vi "ReadPatternFile.vi"(0 "PatternsXMLFileIn":path, 1 "PatternXMLFileContent":string, 5 "error in (no error)":errorcluster) -> (14 "Pattern":T3={"Version"="", "ID"="State", "Name"="State", "Category"="Behavioral", "Help"="State.htm", "Desc"="Allow an object to alter its behavior when its internal state changes. The object will appear to change its class."}, 15 "Nodes":T4[](array[typedef])=[{"ID"="Context", "Type"=enum."Class", "Name"="Context", "Stereotype"="", "X"=0, "Y"=0, "TypeSpecificData"=variant(cluster{"Attributes":cluster{"ID":string, "Name":string}[], "Methods":cluster{"ID":string, "Name":string}[]} {"Attributes"=[{"ID"="StateRef", "Name"="CurrentState : State"}], "Methods"=[{"ID"="Request", "Name"="Request()"}]})}, {"ID"="State", "Type"=enum."Class", "Name"="State", "Stereotype"="ABSTRACT", "X"=0, "Y"=0, "TypeSpecificData"=variant(cluster{"Attributes":cluster{"ID":string, "Name":string}[], "Methods":cluster{"ID":string, "Name":string}[]} {"Attributes"=[], "Methods"=[{"ID"="Handle", "Name"="Handle()"}]})}, {"ID"="ConcreteStateA", "Type"=enum."Class", "Name"="ConcreteStateA", "Stereotype"="", "X"=0, "Y"=0, "TypeSpecificData"=variant(cluster{"Attributes":cluster{"ID":string, "Name":string}[], "Methods":cluster{"ID":string, "Name":string}[]} {"Attributes"=[], "Methods"=[{"ID"="Handle", "Name"="Handle()"}]})}, {"ID"="ConcreteStateB", "Type"=enum."Class", "Name"="ConcreteStateB", "Stereotype"="", "X"=0, "Y"=0, "TypeSpecificData"=variant(cluster{"Attributes":cluster{"ID":string, "Name":string}[], "Methods":cluster{"ID":string, "Name":string}[]} {"Attributes"=[], "Methods"=[{"ID"="Handle", "Name"="Handle()"}]})}, {"ID"="RequestNote", "Type"=enum."Note", "Name"="", "Stereotype"="", "X"=0, "Y"=0, "TypeSpecificData"=variant(cluster{"Text":string, "Links":cluster{"ID":string, "source":string}[]} {"Text"="state->Handle()", "Links"=[{"ID"="ToRequest", "source"="Request"}]})}], 16 "Links":T1[](array[typedef])=[{"ID"="Aggregation", "Type"=enum."Aggregation", "Name"="", "StartText"="state", "EndText"="", "From"="Context", "To"="State"}], 17 "Valid":bool, 19 "error out":errorcluster)   [LabVIEW 2014]
uses:
  <resource>/Framework/Providers/Open_GDS/UML/DesignPattern/SubVIs/DesignPatterns_Node.ctl
  <resource>/Framework/Providers/Open_GDS/UML/DesignPattern/SubVIs/DesignPatterns_NodeType.ctl
  <resource>/Framework/Providers/Open_GDS/UML/DesignPattern/SubVIs/DesignPatterns_Pattern.ctl
  <resource>/Framework/Providers/Open_GDS/UML/DesignPattern/SubVIs/DesignPatterns_Link.ctl
  <resource>/Framework/Providers/Open_GDS/UML/DesignPattern/SubVIs/DesignPatterns_LinkType.ctl
  <resource>/Framework/Providers/Open_GDS/UML/DesignPattern/SubVIs/DesignPatterns_ClassNodeData.ctl
  <resource>/Framework/Providers/Open_GDS/UML/DesignPattern/SubVIs/DesignPatterns_Attribute.ctl
  <resource>/Framework/Providers/Open_GDS/UML/DesignPattern/SubVIs/DesignPatterns_Method.ctl
  <resource>/Framework/Providers/Open_GDS/UML/DesignPattern/SubVIs/DesignPatterns_InterfaceNodeData.ctl
  <resource>/Framework/Providers/Open_GDS/UML/DesignPattern/SubVIs/DesignPatterns_NoteNodeData.ctl
  <resource>/Framework/Providers/Open_GDS/UML/DesignPattern/SubVIs/DesignPatterns_NoteLink.ctl
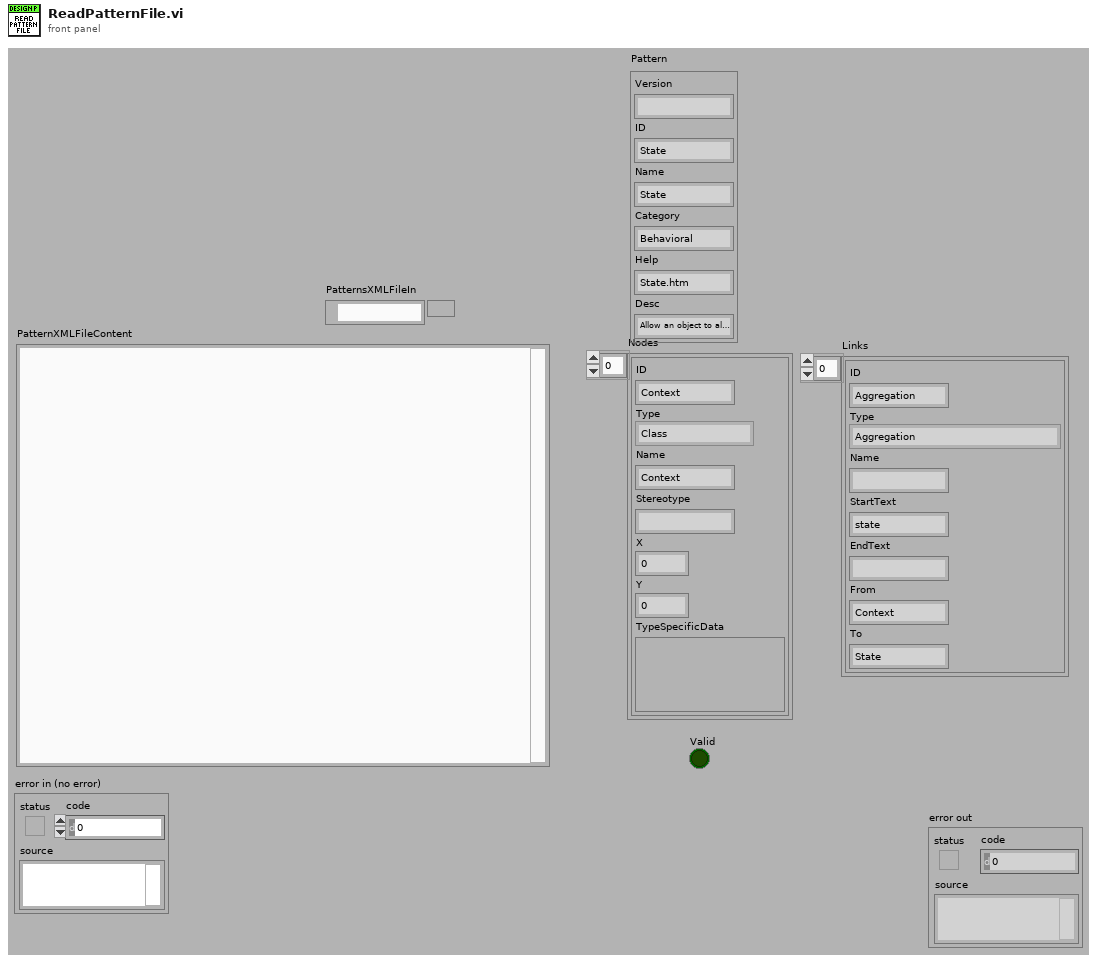
[diagram p1: front panel]
types:
  T1 = typedef "DesignPatterns_Link.ctl" = cluster{"ID":string, "Type":T2, "Name":string, "StartText":string, "EndText":string, "From":string, "To":string}
  T2 = typedef "DesignPatterns_LinkType.ctl" = enum16{"Dependency", "Inheritance", "Interface", "Association", "Aggregation", "CompositeAggregation"}
  T3 = typedef "DesignPatterns_Pattern.ctl" = cluster{"Version":string, "ID":string, "Name":string, "Category":string, "Help":string, "Desc":string}
  T4 = typedef "DesignPatterns_Node.ctl" = cluster{"ID":string, "Type":T5, "Name":string, "Stereotype":string, "X":i32, "Y":i32, "TypeSpecificData":variant}
  T5 = typedef "DesignPatterns_NodeType.ctl" = enum16{"Class", "Interface", "Note", "Package"}
  T6 = cluster{"Text":string, "Valid":bool, "Pattern":T3, "Nodes":T4[], "Links":T1[]}
  T7 = typedef "DesignPatterns_ClassNodeData.ctl" = cluster{"Description":string, "Attributes":T8[], "Methods":T9[]}
  T8 = typedef "DesignPatterns_Attribute.ctl" = cluster{"ID":string, "Name":string}
  T9 = typedef "DesignPatterns_Method.ctl" = cluster{"ID":string, "Name":string}
  T10 = typedef "DesignPatterns_InterfaceNodeData.ctl" = cluster{"Methods":T9[]}
  T11 = typedef "DesignPatterns_NoteNodeData.ctl" = cluster{"Text":string, "Links":T12[]}
  T12 = typedef "DesignPatterns_NoteLink.ctl" = cluster{"ID":string, "source":string}
  T13 = cluster{"id":string, "node.type":T5, "link.type":T2, "name":string, "stereotype":string, "X":i32, "Y":i32, "starttext":string, "endtext":string, "from":string, "to":string, "version":string, "category":string, "help":string}
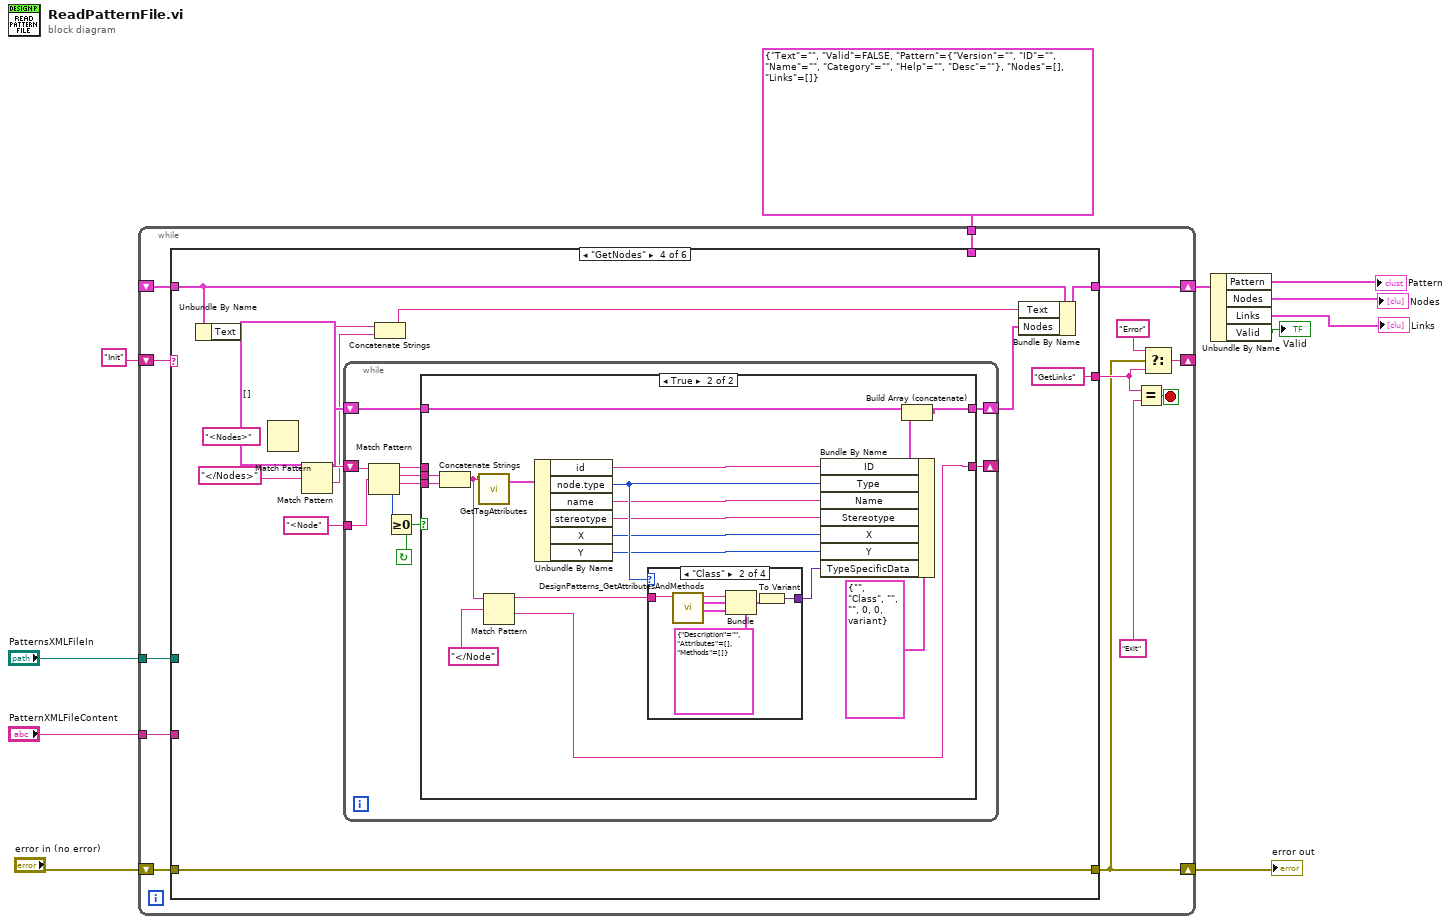
[diagram p0: block diagram]
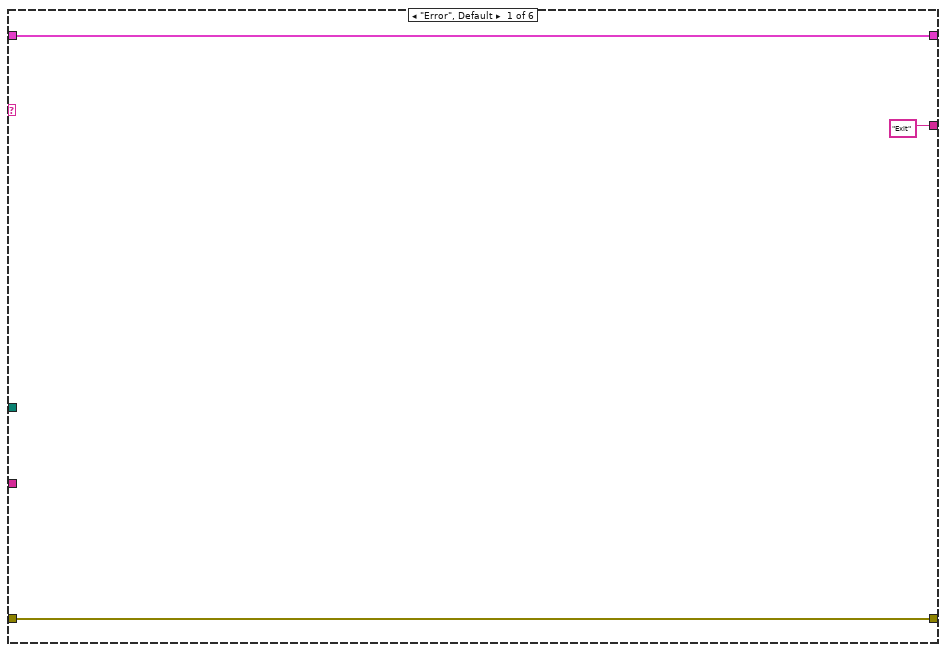
[diagram p2: hidden frame]
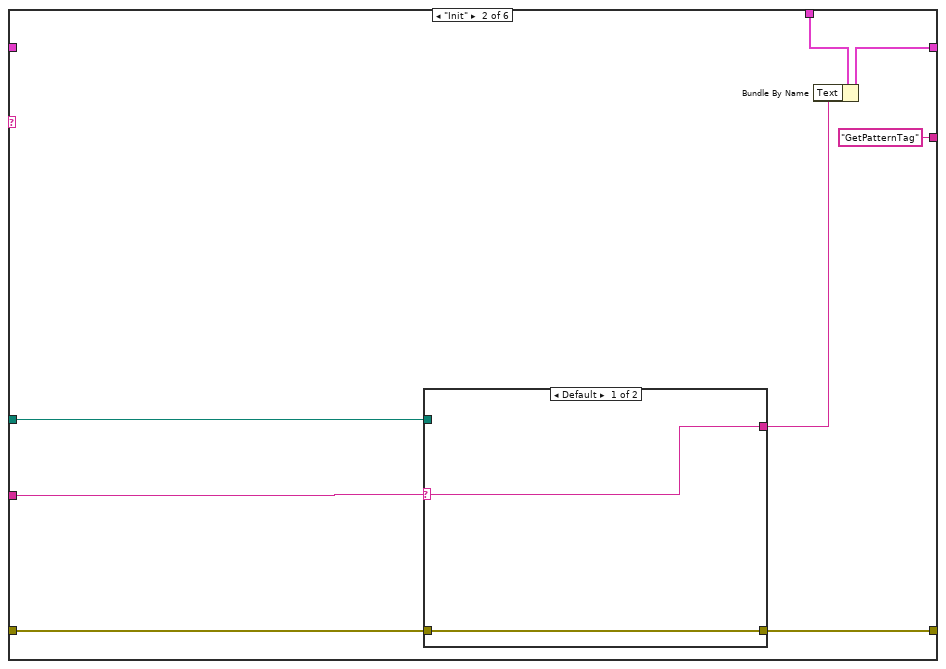
[diagram p3: hidden frame]
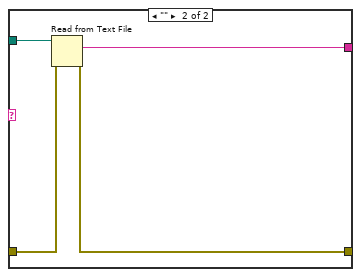
[diagram p4: hidden frame]
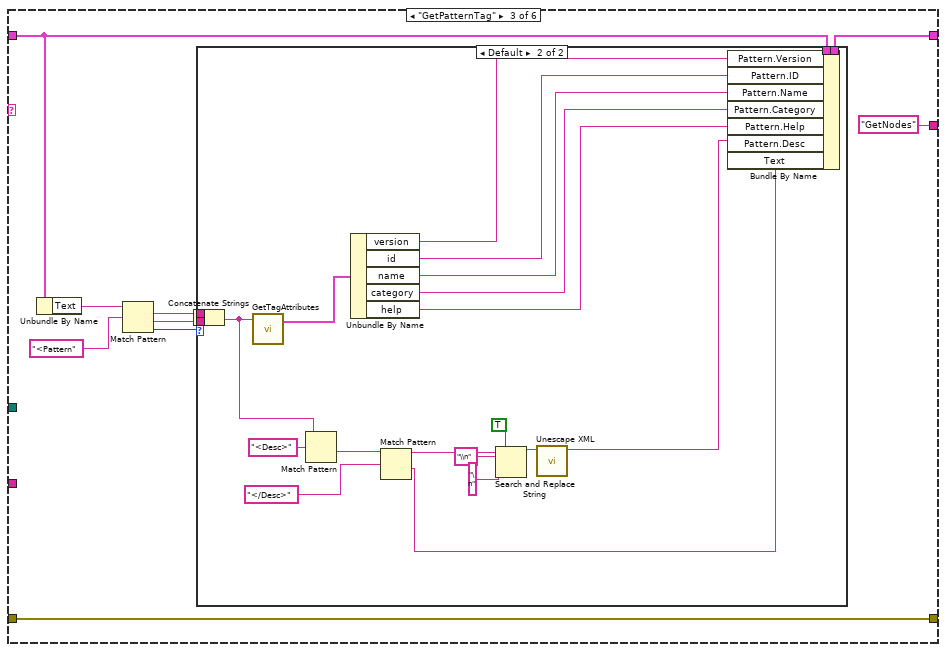
[diagram p5: hidden frame]
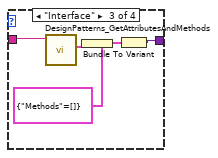
[diagram p9: hidden frame]
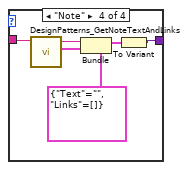
[diagram p10: hidden frame]
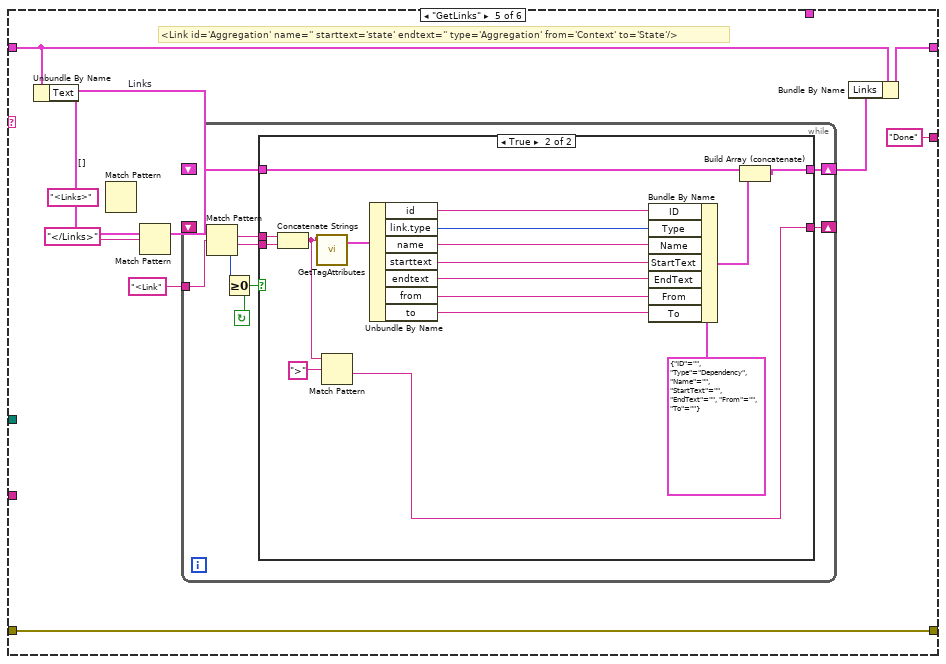
[diagram p11: hidden frame]
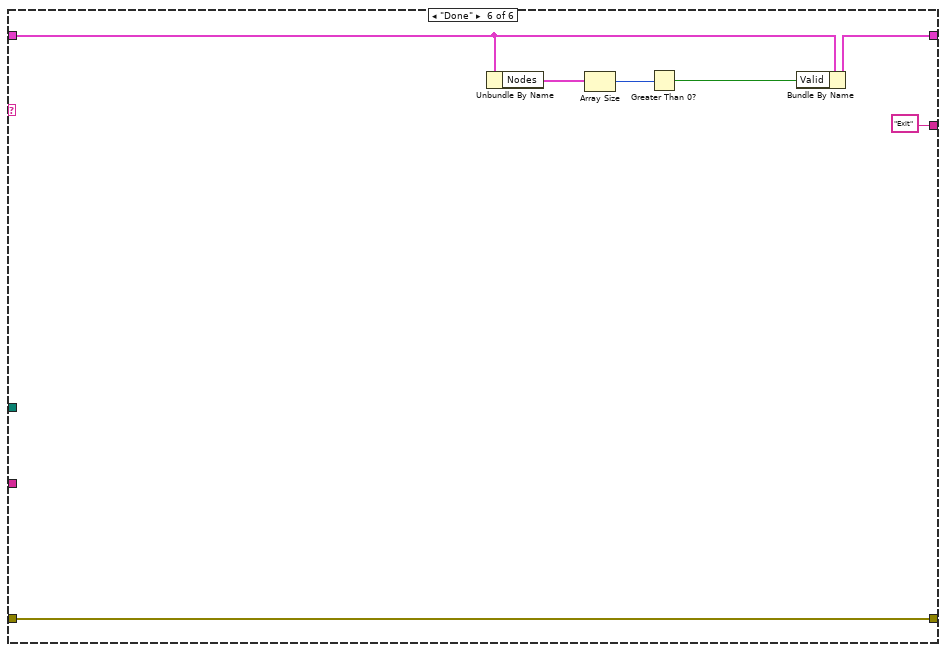
[diagram p13: hidden frame]
diagram:
  n1 = while {
    shift-right: [w17] -> w8
    shift-left: "error in (no error)" -> [w24]
    shift-right: [w22] -> _
    shift-left: "Init" -> [w23]
    shift-right: [w16] -> w11
    shift-left: _ -> [w15]
    tunnel: "PatternsXMLFileIn" -> [w14]
    tunnel: "PatternXMLFileContent" -> [w13]
    tunnel: T6 {"Text"="", "Valid"=FALSE, "Pattern"={"Version"="", "ID"="", "Name"="", "Category"="", "Help"="", "Desc"=""}, "Nodes"=[], "Links"=[]} -> [w12]
    stop <- w21 stop-if-true
    n2 = case shown="\"GetNodes\"" w23 {
      tunnel: w24 -> [w27 w32 w49 w87 w146 w174]
      tunnel: [w27 w31 w49 w87 w146 w174] -> w17
      tunnel: ["Exit" "GetPatternTag" "GetNodes" "GetLinks" "Done" "Exit"] -> w18
      tunnel: [w25 w29 w48 w79 w138 w180] -> w16
      tunnel: w15 -> [w25 _ w47 w80 w139 w179]
      tunnel: w14 -> [_ w33 _ _ _ _]
      tunnel: w13 -> [_ w34 _ _ _ _]
      tunnel: w12 -> [_ w30 _ _ _ _]
      frame "Error", Default {
      }
      frame "Init" {
        n3 = case shown="Default" w34 {
          selector: w34 -> [w36 _]
          tunnel: w33 -> [_ w41]
          tunnel: w32 -> [w37 w40]
          tunnel: [w37 w39] -> w31
          tunnel: [w36 w38] -> w28
          frame Default {
          }
          frame "" {
            n4 = Read from Text File(file (use dialog)=w41, error in=w40) -> (text=w38:string, error out=w39:errorcluster)  [unwired: 4 out]
          }
        }
        n5 = Bundle By Name(cluster=w30, "Text"=w28) -> (w29:T6)
      }
      frame "GetPatternTag" {
        n6 = Unbundle By Name(w47) -> ("Text"=w46:string)
        n7 = Match Pattern(string=w46, regular expression="<Pattern") -> (match substring=w44:string, after substring=w43:string, offset past match=w42:i32)  [unwired: 2 out]
        n8 = case shown="Default" w42 {
          tunnel: [w51 w72] -> w48
          tunnel: w47 -> [w51 w71]
          tunnel: w44 -> [_ w70]
          tunnel: w43 -> [_ w69]
          frame -1 {
          }
          frame Default {
            n9 = Concatenate Strings(w70, w69) -> (w58:string)
            n10 = call <resource>:"GetTagAttributes.vi"("TextIn"=w58) -> ("Attributes"=w57:T13)  [unwired: 18 out]
            n11 = Match Pattern(string=w58, regular expression="<Desc>") -> (after substring=w67:string)  [unwired: 4 out]
            n12 = Unbundle By Name(w57) -> ("version"=w56:string, "id"=w55:string, "name"=w54:string, "category"=w53:string, "help"=w52:string)
            n13 = Match Pattern(string=w67, regular expression="</Desc>") -> (before substring=w65:string, after substring=w59:string)  [unwired: 3 out]
            n14 = Search and Replace String(replace all?=TRUE ("replace all? (F)"), input string=w65, search string="\\n", replace string="\n" ("replace string (\"\")")) -> (result string=w61:string)  [unwired: 1 in, 6 out]
            n15 = call <vilib>:"Unescape XML.vi"("XML String In"=w61) -> ("XML String Out"=w60:string)  [unwired: 1 in, 9 out]
            n16 = Bundle By Name(cluster=w71, "Pattern.Version"=w56, "Pattern.ID"=w55, "Pattern.Name"=w54, "Pattern.Category"=w53, "Pattern.Help"=w52, "Pattern.Desc"=w60, "Text"=w59) -> (w72:T6)
          }
        }
      }
      frame "GetNodes" {
        n17 = Unbundle By Name(w80) -> ("Text"=w85:string)
        n18 = Match Pattern(string=w85, regular expression="<Nodes>") -> (before substring=w75:string, after substring=w84:string)  [unwired: 3 out]
        n19 = Match Pattern(string=w84, regular expression="</Nodes>") -> (before substring=w82:string, after substring=w74:string)  [unwired: 3 out]
        n20 = while {
          shift-right: [w91] -> _
          shift-left: w82 -> [w95]
          tunnel: "<Node" ("regular expression") -> [w94]
          shift-right: [w89] -> w77
          shift-left: T4[] [] -> [w90]
          stop <- w92 continue-if-true
          n21 = Match Pattern(string=w95, regular expression=w94) -> (before substring=w88:string, match substring=w96:string, after substring=w97:string, offset past match=w93:i32)  [unwired: 1 out]
          n22 = Greater Or Equal To 0?(x=w93) -> (x >= 0?=w92:bool)
          n23 = case shown="True" w92 {
            tunnel: w97 -> [_ w116]
            tunnel: w96 -> [_ w115]
            tunnel: [_ w106] -> w91
            tunnel: w90 -> [w98 w113]
            tunnel: [w98 w112] -> w89
            tunnel: w88 -> [_ _]
            frame False {
            }
            frame True {
              n24 = Concatenate Strings(w115, w116) -> (w107:string)
              n25 = call <resource>:"GetTagAttributes.vi"("TextIn"=w107) -> ("Attributes"=w105:T13)  [unwired: 18 out]
              n26 = Match Pattern(string=w107, regular expression="</Node") -> (before substring=w108:string, after substring=w106:string)  [unwired: 3 out]
              n27 = Unbundle By Name(w105) -> ("id"=w104:string, "node.type"=w103:T5, "name"=w102:string, "stereotype"=w101:string, "X"=w100:i32, "Y"=w99:i32)
              n28 = case shown="\"Class\"" w103 {
                tunnel: w108 -> [_ w118 w124 w132]
                tunnel: [_ w119 w125 w133] -> w110
                frame Default {
                }
                frame "Class" {
                  n29 = call <resource>:"DesignPatterns_GetAttributesAndMethods.vi"("ClassText"=w118) -> ("Methods"=w117:T9[], "Attributes"=w122:T8[], "Desciption"=w123:string)  [unwired: 8 out]
                  n30 = Bundle(cluster=T7 {"Description"="", "Attributes"=[], "Methods"=[]}, "Description"=w123, "Attributes"=w122, "Methods"=w117) -> (w121:T7)
                  n31 = To Variant(anything=w121) -> (Variant=w119:variant)
                }
                frame "Interface" {
                  n32 = call <resource>:"DesignPatterns_GetAttributesAndMethods.vi"("ClassText"=w124) -> ("Attributes"=w127:T8[])  [unwired: 10 out]
                  n33 = Bundle(cluster=T10 {"Methods"=[]} ("ClassSpecificData"), "Methods"=w127) -> (w126:T10)
                  n34 = To Variant(anything=w126) -> (Variant=w125:variant)
                }
                frame "Note" {
                  n35 = call <resource>:"DesignPatterns_GetNoteTextAndLinks.vi"("ClassText"=w132) -> ("Links"=w129:T12[], "Text"=w130:string)  [unwired: 9 out]
                  n36 = Bundle(cluster=T11 {"Text"="", "Links"=[]} ("Link"), "Text"=w130, "Links"=w129) -> (w134:T11)
                  n37 = To Variant(anything=w134) -> (Variant=w133:variant)
                }
              }
              n38 = Bundle By Name(cluster=T4 {"ID"="", "Type"=enum."Class", "Name"="", "Stereotype"="", "X"=0, "Y"=0, "TypeSpecificData"=variant} ("Class"), "ID"=w104, "Type"=w103, "Name"=w102, "Stereotype"=w101, "X"=w100, "Y"=w99, "TypeSpecificData"=w110) -> (w111:T4)
              n39 = Build Array (concatenate)(w113, w111) -> (w112:T4[])
            }
          }
        }
        n40 = Concatenate Strings(w75, w74) -> (w73:string)
        n41 = Bundle By Name(cluster=w80, "Text"=w73, "Nodes"=w77) -> (w79:T6)
      }
      frame "GetLinks" {
        w137 = T1[] []  # Links
        # "<Link id='Aggregation' name='' starttext='state' endtext='' type='Aggregation' from='Context' to='State'/>"
        n42 = Unbundle By Name(w139) -> ("Text"=w144:string)
        n43 = Match Pattern(string=w144, regular expression="<Links>") -> (after substring=w143:string)  [unwired: 4 out]
        n44 = Match Pattern(string=w143, regular expression="</Links>") -> (before substring=w141:string)  [unwired: 4 out]
        n45 = while {
          shift-right: [w149] -> _
          shift-left: w141 -> [w153]
          tunnel: "<Link" ("regular expression") -> [w152]
          shift-right: [w147] -> w136
          shift-left: w137 -> [w148]
          stop <- w150 continue-if-true
          n46 = Match Pattern(string=w153, regular expression=w152) -> (match substring=w154:string, after substring=w155:string, offset past match=w151:i32)  [unwired: 2 out]
          n47 = Greater Or Equal To 0?(x=w151) -> (x >= 0?=w150:bool)
          n48 = case shown="True" w150 {
            tunnel: w155 -> [_ w173]
            tunnel: w154 -> [_ w172]
            tunnel: [_ w166] -> w149
            tunnel: w148 -> [w156 w171]
            tunnel: [w156 w170] -> w147
            frame False {
            }
            frame True {
              n49 = Concatenate Strings(w172, w173) -> (w167:string)
              n50 = call <resource>:"GetTagAttributes.vi"("TextIn"=w167) -> ("Attributes"=w165:T13)  [unwired: 18 out]
              n51 = Match Pattern(string=w167, regular expression=">") -> (after substring=w166:string)  [unwired: 4 out]
              n52 = Unbundle By Name(w165) -> ("id"=w163:string, "link.type"=w162:T2, "name"=w161:string, "starttext"=w160:string, "endtext"=w159:string, "from"=w158:string, "to"=w157:string)
              n53 = Bundle By Name(cluster=T1 {"ID"="", "Type"=enum."Dependency", "Name"="", "StartText"="", "EndText"="", "From"="", "To"=""} ("Node"), "ID"=w163, "Type"=w162, "Name"=w161, "StartText"=w160, "EndText"=w159, "From"=w158, "To"=w157) -> (w169:T1)
              n54 = Build Array (concatenate)(w171, w169) -> (w170:T1[])
            }
          }
        }
        n55 = Bundle By Name(cluster=w139, "Links"=w136) -> (w138:T6)
      }
      frame "Done" {
        n56 = Unbundle By Name(w179) -> ("Nodes"=w178:T4[])
        n57 = Array Size(array=w178) -> (size(s)=w177:i32)
        n58 = Greater Than 0?(x=w177) -> (x > 0?=w176:bool)
        n59 = Bundle By Name(cluster=w179, "Valid"=w176) -> (w180:T6)
      }
    }
    n60 = Equal?(x=w18, y="Exit") -> (x = y?=w21:bool)
    n61 = Select(t="Error", s=w17, f=w18) -> (s? t:f=w22:string)
  }
  "error out" <- w8
  n62 = Unbundle By Name(w11) -> ("Pattern"=→"Pattern":T3, "Nodes"=→"Nodes":T4[], "Links"=→"Links":T1[], "Valid"=→"Valid":bool)
